vi "computeAlpha.vi"(8 "error in (no error)":errorcluster, 11 "LaguerreDeconClass in":refnum<class "LaguerreDeconEngineClass.lvclass">) -> (0 "error out":errorcluster, 3 "LaguerreDeconClass out":refnum<class "LaguerreDeconEngineClass.lvclass">)   [LabVIEW 2020, in "LaguerreDeconEngineClass.lvclass"]
uses:
  LaguerreDeconEngineClass.lvclass
  LaguerreDeconEngineClass.lvclass/LaguerreDeconEngineClass.ctl
  LaguerreDeconLib.lvlib
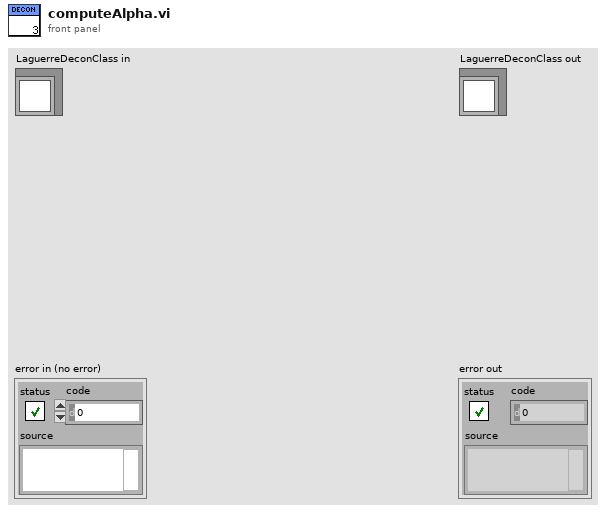
[diagram p1: front panel]
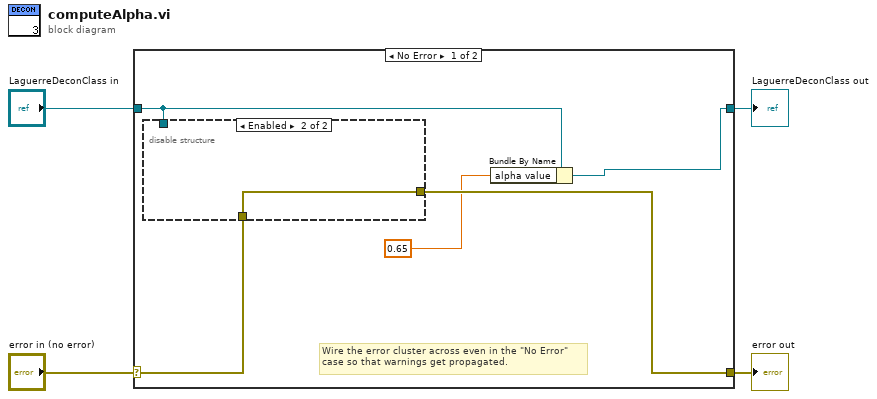
[diagram p0: block diagram]
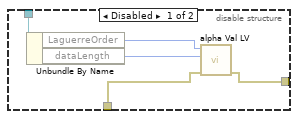
[diagram p2: hidden frame]
diagram:
  n1 = case shown="No Error" "error in (no error)" {
    selector: "error in (no error)" -> [w7 w17]
    tunnel: [w6 w17] -> w3
    tunnel: [w8 w16] -> w1
    tunnel: "LaguerreDeconClass in" -> [w9 w16]
    frame No Error {
      # "Wire the error cluster across even in the \"No Error\"\ncase so that warnings get propagated."
      n2 = disable-structure shown="Enabled" {
        disable-tunnel: w9 -> [w12 _]
        disable-tunnel: w7 -> [w11 w15]
        disable-tunnel: [w10 w15] -> w6
        frame Disabled {
          n3 = Unbundle By Name(w12) -> ("LaguerreOrder"=w14:u32, "dataLength"=w13:u32)
          n4 = call "alpha Val LV.vi"("error in (no error)"=w11, "dataLength"=w13, "laguerreOrder"=w14) -> ("error out"=w10:errorcluster)  [unwired: 7 in, 1 out]
        }
        frame Enabled {
        }
      }
      n5 = Bundle By Name(cluster=w9, "alpha value"=0.65) -> (w8:refnum<class "LaguerreDeconEngineClass.lvclass">)
    }
    frame Error {
    }
  }
  "error out" <- w3
  "LaguerreDeconClass out" <- w1
